vi "Wait.vi"(2 "milliseconds to wait":u32, 3 "Stimulator":T1={"Stim Open Data"={"Name"="", "Mode"=enum."LIVE", "Visa Timeout"=0}, "Stim Init Data"={"Frequency"=0.0, "N Factor"=0, "D/T Int"=0.0, "Active Channels"=[], "LF Channels"=[]}, "Stim Update Data"={"Pulse Mode"=[enum."Single"], "Current"=[], "Pulse Dur"=[]}, "Stim Status"={"Open"=FALSE, "On"=FALSE}}) -> (0 "Milliseconds Waited":u32, 1 "Stimulator":T1={"Stim Open Data"={"Name"="", "Mode"=enum."LIVE", "Visa Timeout"=0}, "Stim Init Data"={"Frequency"=0.0, "N Factor"=0, "D/T Int"=0.0, "Active Channels"=[], "LF Channels"=[]}, "Stim Update Data"={"Pulse Mode"=[enum."Single"], "Current"=[], "Pulse Dur"=[]}, "Stim Status"={"Open"=FALSE, "On"=FALSE}})   [LabVIEW 2019]
uses:
  Version 2/Data Type Defs/Stimulator.ctl
  Version 2/Data Type Defs/Stim Open Data.ctl
  Version 2/Data Type Defs/Stim Init Data.ctl
  Version 2/Data Type Defs/Stim Update Data.ctl
  Version 2/Data Type Defs/Pulse Mode (array).ctl
  Version 2/Data Type Defs/Stim Status.ctl
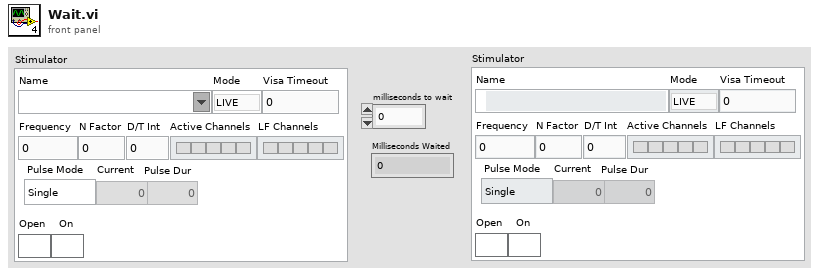
[diagram p1: front panel]
types:
  T1 = typedef "Stimulator.ctl" = cluster{"Stim Open Data":T2, "Stim Init Data":T3, "Stim Update Data":T4, "Stim Status":T6}
  T2 = typedef "Stim Open Data.ctl" = cluster{"Name":refnum<visa-resource-name>, "Mode":enum16{"LIVE", "SIM"}, "Visa Timeout":u32}
  T3 = typedef "Stim Init Data.ctl" = cluster{"Frequency":dbl, "N Factor":u8, "D/T Int":dbl, "Active Channels":bool[], "LF Channels":bool[]}
  T4 = typedef "Stim Update Data.ctl" = cluster{"Pulse Mode":T5, "Current":u32[], "Pulse Dur":u32[]}
  T5 = typedef "Pulse Mode (array).ctl" = enum16{"Single", "Doublet", "Triplet"}[]
  T6 = typedef "Stim Status.ctl" = cluster{"Open":bool, "On":bool}
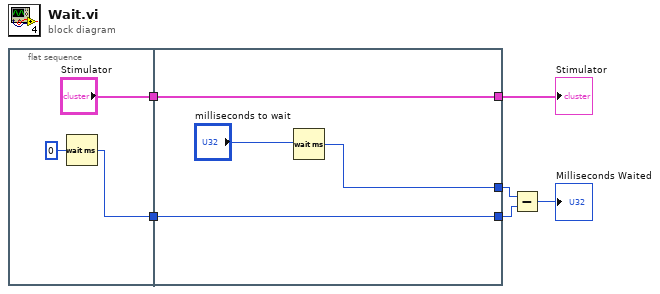
[diagram p0: block diagram]
diagram:
  n1 = flat-sequence {
    tunnel: [w8] -> w6
    tunnel: ["Stimulator"] -> w2
    tunnel: [w12] -> w5
    tunnel: [w11] -> w4
    tunnel: w6 -> [w11]
    tunnel: w2 -> [w10]
    tunnel: [w10] -> w1
    frame #0 {
      n2 = Wait (ms)(milliseconds to wait=u32 0) -> (millisecond timer value=w8:u32)
    }
    frame #1 {
      n3 = Wait (ms)(milliseconds to wait="milliseconds to wait") -> (millisecond timer value=w12:u32)
    }
  }
  n4 = Subtract(x=w5, y=w4) -> (x-y=→"Milliseconds Waited":u32)
  "Stimulator" <- w1
